vi "Benchmark FIFO Output.vi"(6 "timed out?":bool, 8 "error in (no error)":errorcluster, 9 "T_Out":i64, 10 "T_Write":i64, 11 "CIFCorePlugin in":refnum<class "CIFCorePlugin.lvclass">) -> (0 "error out":errorcluster, 3 "CIFCorePlugin out":refnum<class "CIFCorePlugin.lvclass">)   [LabVIEW 2021, in "CIFCorePlugin.lvclass"]
doc: "This will track the statistics for the output error (the actual time of the output compared to the target T_Out).\n\nBy default it is automatically called in \"Timestamp T_Out Control.vi\", inside \"Sleep for T_Out.VI\" with the assumption that the write function latency is immaterial and difficult to measure precisely. However It can be disabled in that VI and instead called directly after the IO write function for user controlled timestamps."
uses:
  CIFCorePlugin.lvclass
  CIFCorePlugin.lvclass/CIFCorePlugin.ctl
  <vilib>/CIF Foundation/CIF Utilities/Statistics/I64/Stats_I64_CIF_U.lvclass/Stats_I64_CIF_U.ctl
  <vilib>/CIF Foundation/CIF Utilities/Time/System Time/LabVIEW Time to TAI Time.vi
  <vilib>/CIF Foundation/CIF Utilities/Statistics/I64/X1 minus X0.vi/dfabcf33-0dbc-4041-80a5-3dc0c86d2989.vi
  <vilib>/CIF Foundation/CIF Utilities/Statistics/I64/X1 minus X0.vi/dfabcf33-0dbc-4041-80a5-3dc0c86d2989.vi/9eb60a9a-770f-4d2d-8b3f-8465c267ecc9.vi
  <vilib>/CIF Foundation/CIF Utilities/Statistics/I64/Stats_I64_CIF_U.lvclass
  <vilib>/CIF Foundation/CIF Utilities/Time/Time_CIF_U.lvlib
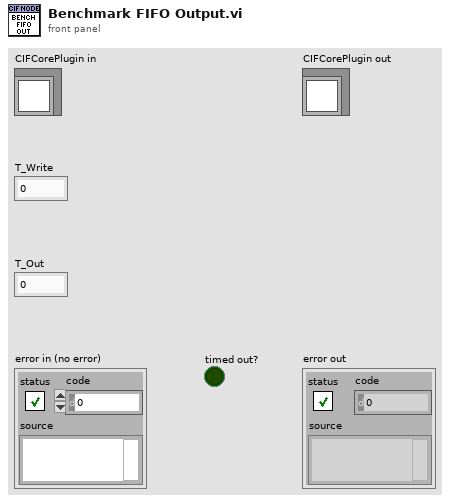
[diagram p1: front panel]
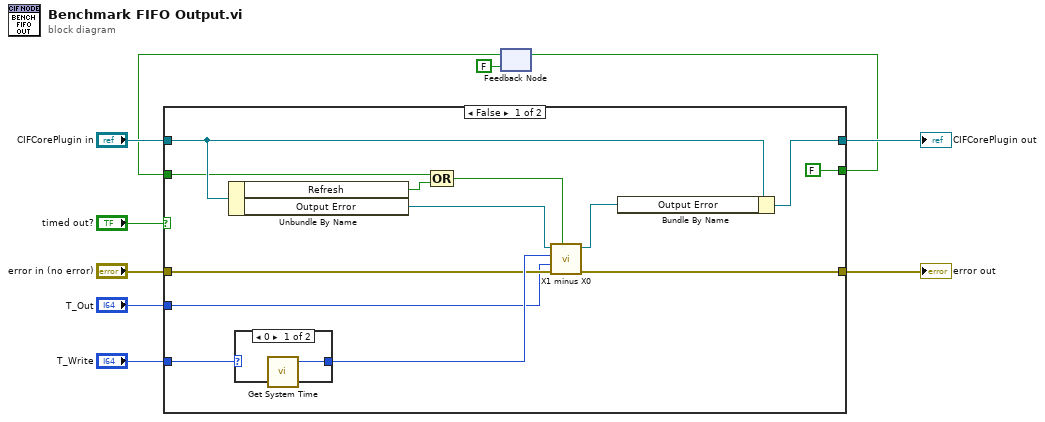
[diagram p0: block diagram]
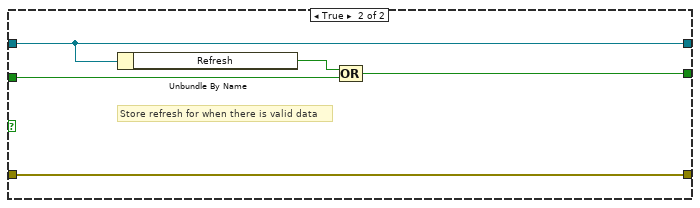
[diagram p3: hidden frame]
diagram:
  n1 = feedback #1(FALSE ("Refresh")) -> (w1:bool)
  n2 = case shown="False" "timed out?" {
    tunnel: [w17 w30] -> w10
    tunnel: [w22 w29] -> w8
    tunnel: "CIFCorePlugin in" -> [w23 w29]
    tunnel: "T_Out" -> [w15 _]
    tunnel: "T_Write" -> [w21 _]
    tunnel: "error in (no error)" -> [w16 w30]
    tunnel: [FALSE w26] -> w3
    tunnel: w1 -> [w13 w28]
    frame False {
      n3 = Unbundle By Name(w23) -> ("Refresh"=w12:bool, "Output Error"=w20:refnum<class "Stats_I64_CIF_U.lvclass">)
      n4 = case shown="0" w21 {
        selector: w21 -> [_ w25]
        tunnel: [w24 w25] -> w19
        frame 0 {
          n5 = call <vilib>:"Get System Time.vi"() -> ("Time (ns)"=w24:i64)  [unwired: 5 in]
        }
        frame 1, Default {
        }
      }
      n6 = Compound Arithmetic op=OR(w13, w12) -> (w11:bool)
      n7 = call <vilib>:"X1 minus X0.vi"("Reinit"=w11, "error in (no error)"=w16, "X0"=w15, "X1"=w19, "Stats_I64_CIF_U in"=w20) -> ("error out"=w17:errorcluster, "Stats_I64_CIF_U out"=w18:refnum<class "Stats_I64_CIF_U.lvclass">)  [unwired: 5 in]
      n8 = Bundle By Name(cluster=w23, "Output Error"=w18) -> (w22:refnum<class "CIFCorePlugin.lvclass">)
    }
    frame True {
      # "Store refresh for when there is valid data"
      n9 = Unbundle By Name(w29) -> ("Refresh"=w27:bool)
      n10 = Compound Arithmetic op=OR(w27, w28) -> (w26:bool)
    }
  }
  "error out" <- w10
  "CIFCorePlugin out" <- w8
  n11 = feedback-in #1(w3) -> ()
